vi "main.vi"() -> ()   [LabVIEW 2022 SP3]
uses:
  <vilib>/Instr/_visa.llb/VISA Configure Serial Port (Instr).vi
panel:
  out "ENC初始值":u16
  out "无符号字节数组":u8[](array[numeric])
  out "读取缓冲区":string
  in  "kd2":dbl
  in  "ki2":dbl
  in  "kp2":dbl
  in  "kd1":dbl
  in  "ki1":dbl
  in  "kp1":dbl
  in  "目标ADC":dbl
  out "ENC":u16(graph)
  out "ADC":u16(graph)
  in  "匀速转动":bool
  in  "启动":bool
  out "ENC":u16
  out "ADC":u16
  in  "停止":bool
  in  "终止符":u8=10 caption="终止符\n(0xA = '\\n' = LF)" format="%.0x"
  in  "数据比特":u16(ring)=10 caption="停止位（10: 1位）" items=["1.0"=10, "1.5"=15, "2.0"=20]
  in  "data bits (8)":u16=8 caption="数据比特(8)" min=5 max=8 step=1
  in  "启用终止符":bool=TRUE caption="启用终止符 (T)"
  in  "奇偶":enum16{"None", "Odd", "Even", "Mark", "Space"}(ring) caption="奇偶（0:无）"
  in  "baud rate (9600)":u32=9600 caption="波特率(9600)"
  in  "端口":refnum<visa-resource-name> caption="VISA资源名称"
  # "仪表盘"
  # "串口调试"
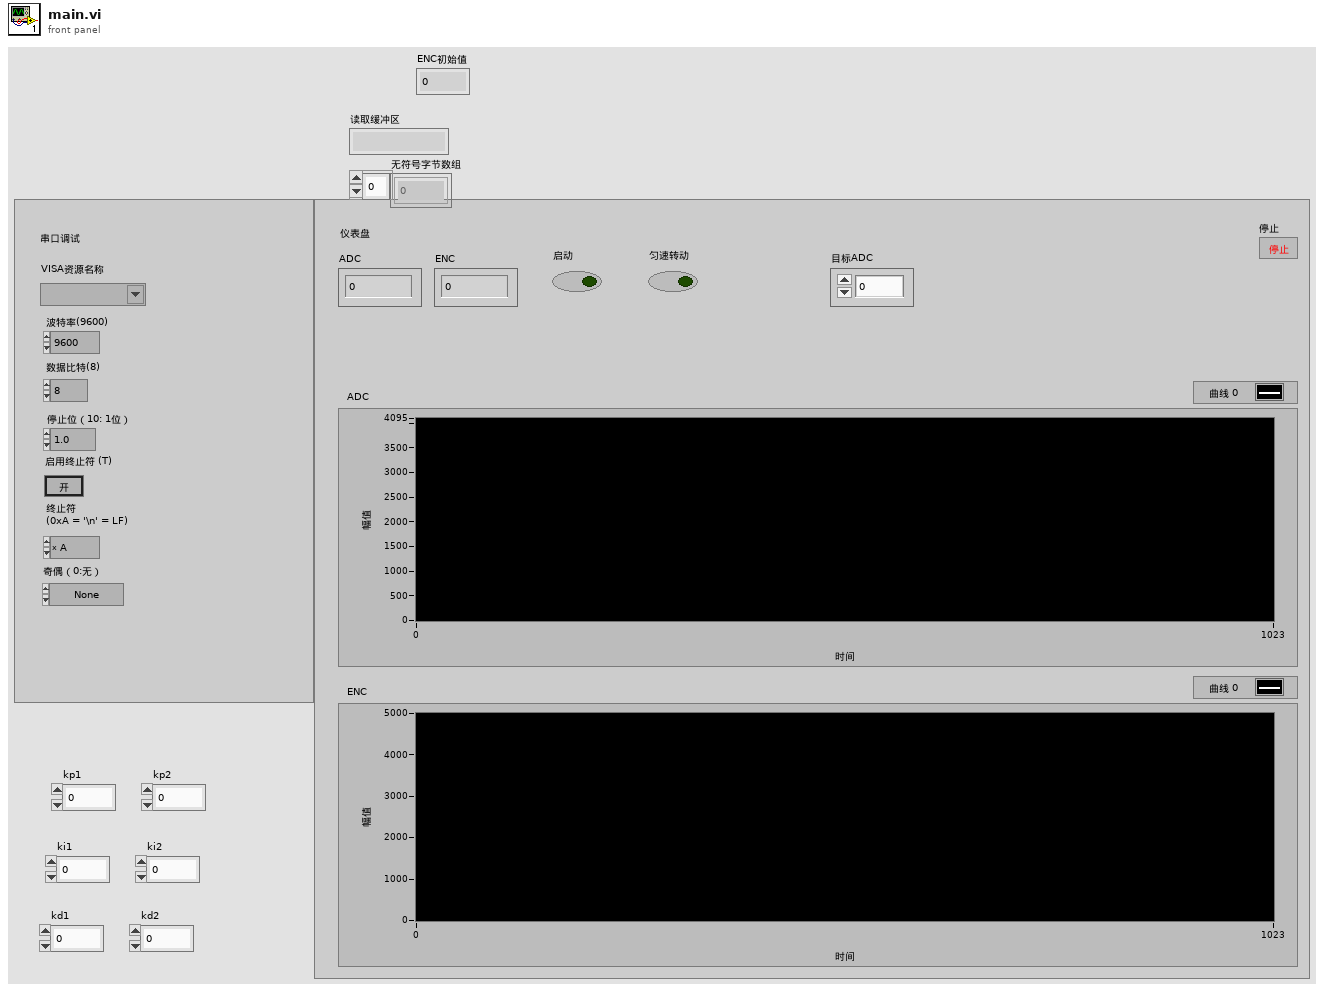
[diagram p1: front panel]
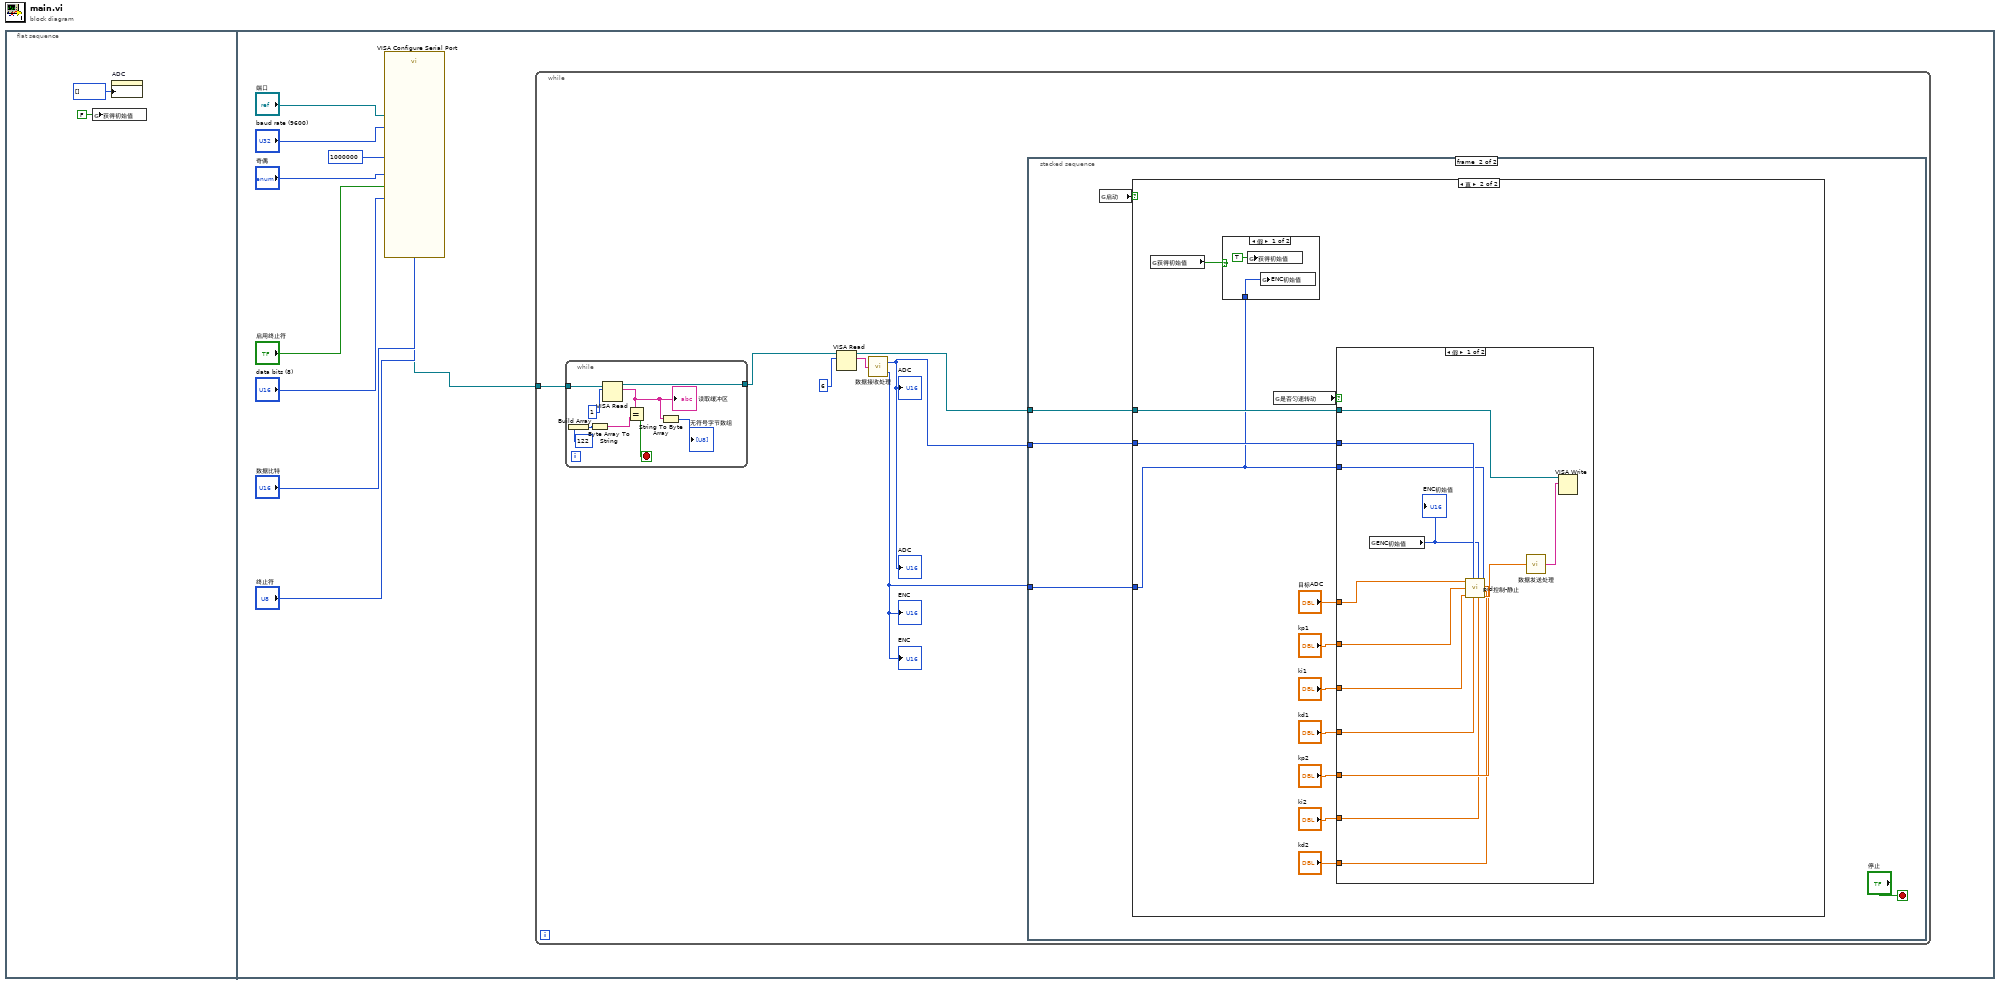
[diagram p0: block diagram]
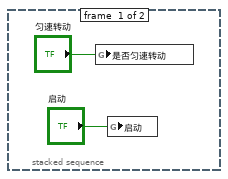
[diagram p2: hidden frame]
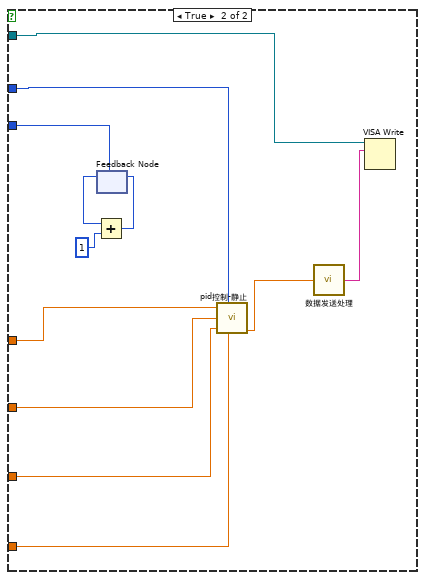
[diagram p5: hidden frame]
diagram:
  n1 = flat-sequence {
    frame #0 {
      n2 = global write "全局 1.vi" "获得初始值"(FALSE ("获得初始值")) -> ()
      n3 = property on="ADC" class="WFChart (严格)"("History Data"=u16[] [] ("历史数据")) -> ()  [unwired: 2 in, 2 out]
    }
    frame #1 {
      n4 = call-poly "VISA Configure Serial Port"("VISA resource name"="端口", "timeout (10sec)"=u32 1000000, "termination char\n(0xA = '\\n' = LF)"="终止符", "Enable Termination\nChar (T)"="启用终止符", "baud rate (9600)"="baud rate (9600)", "data bits (8)"="data bits (8)", "parity (0:none)"="奇偶", "stop bits (10: 1 bit)"="数据比特") -> ("VISA resource name out"=w3:refnum<visa-resource-name>)  [unwired: 6 in, 1 out]
      n5 = while {
        tunnel: w3 -> [w13]
        stop <- "停止" stop-if-true
        n6 = while {
          tunnel: w13 -> [w28]
          tunnel: [w22] -> w12
          stop <- w23 stop-if-true
          n7 = Build Array(u8 122) -> (w25:u8[])
          n8 = Byte Array To String(unsigned byte array=w25) -> (string=w24:string)
          n9 = VISA Read(VISA resource name=w28, byte count=u32 1 ("字节总数")) -> (VISA resource name out=w22:refnum<visa-resource-name>, read buffer=w21:string)  [unwired: 1 in, 2 out]
          "读取缓冲区" <- w21
          n10 = Equal?(x=w21, y=w24) -> (x = y?=w23:bool)
          n11 = String To Byte Array(string=w21) -> (unsigned byte array=→"无符号字节数组":u8[])
        }
        n12 = VISA Read(VISA resource name=w12, byte count=u32 6 ("字节总数")) -> (VISA resource name out=w18:refnum<visa-resource-name>, read buffer=w17:string)  [unwired: 1 in, 2 out]
        n13 = call "数据接收处理.vi"("字符串"=w17) -> ("ADC"=w16:u16, "ENC"=w15:u16)
        "ADC" <- w16
        "ENC" <- w15
        "ADC" <- w16
        "ENC" <- w15
        n14 = stacked-sequence {
          tunnel: w18 -> [_ w31]
          tunnel: w16 -> [_ w34]
          tunnel: w15 -> [_ w33]
          frame #0 {
            n15 = global write "全局 1.vi" "是否匀速转动"("匀速转动") -> ()
            n16 = global write "全局 1.vi" "启动"("启动") -> ()
          }
          frame #1 {
            n17 = global read "全局 1.vi" "启动"() -> (w32:bool)
            n18 = case shown="真" w32 {
              tunnel: w31 -> [_ w44]
              tunnel: w34 -> [_ w45]
              tunnel: w33 -> [_ w35]
              frame False {
              }
              frame True {
                n19 = global read "全局 1.vi" "获得初始值"() -> (w36:bool)
                n20 = case shown="假" w36 {
                  tunnel: w35 -> [w47 _]
                  frame False {
                    n21 = global write "全局 1.vi" "获得初始值"(TRUE ("获得初始值")) -> ()
                    n22 = global write "全局 1.vi" "ENC初始值"(w47) -> ()
                  }
                  frame True {
                  }
                }
                n23 = global read "全局 1.vi" "是否匀速转动"() -> (w46:bool)
                n24 = case shown="假" w46 {
                  tunnel: w45 -> [w58 w70]
                  tunnel: w35 -> [w53 w65]
                  tunnel: w44 -> [w59 w71]
                  tunnel: "ki2" -> [w50 _]
                  tunnel: "ki1" -> [w57 w67]
                  tunnel: "kp1" -> [w56 w68]
                  tunnel: "kp2" -> [w51 _]
                  tunnel: "kd2" -> [w49 _]
                  tunnel: "kd1" -> [w55 w66]
                  tunnel: "目标ADC" -> [w54 w69]
                  frame False {
                    n25 = global read "全局 1.vi" "ENC初始值"() -> (w52:u16)
                    "ENC初始值" <- w52
                    n26 = call "pid控制-静止.vi"("目标p1"=w54, "当前p1"=w58, "kp1"=w56, "ki1"=w57, "kd1"=w55, "目标p2"=w52, "当前p2"=w53, "kp2"=w51, "ki2"=w50, "kd2"=w49) -> ("输出v"=w60:dbl)
                    n27 = call "数据发送处理.vi"("PWM"=w60) -> ("out"=w61:string)
                    n28 = VISA Write(VISA resource name=w59, write buffer=w61) -> ()  [unwired: 1 in, 3 out]
                  }
                  frame True {
                    n29 = feedback #1(w65) -> (w64:u16)
                    n30 = Add(x=w64, y=u16 1) -> (x+y=w62:u16)
                    n31 = feedback-in #1(w62) -> ()
                    n32 = call "pid控制-静止.vi"("目标p1"=w69, "当前p1"=w70, "kp1"=w68, "ki1"=w67, "kd1"=w66) -> ("输出v"=w73:dbl)  [unwired: 5 in]
                    n33 = call "数据发送处理.vi"("PWM"=w73) -> ("out"=w72:string)
                    n34 = VISA Write(VISA resource name=w71, write buffer=w72) -> ()  [unwired: 1 in, 3 out]
                  }
                }
              }
            }
          }
        }
      }
    }
  }
